vi "SaveConfig.vi"(8 "error in (no error)":errorcluster, 11 "DataLogger in":refnum<class "DataLogger.lvclass">) -> (0 "error out":errorcluster, 3 "DataLogger out":refnum<class "DataLogger.lvclass">)   [LabVIEW 2020, in "DataLogger.lvlib" / "DataLogger.lvclass"]
uses:
  DataLogger.lvclass
  DataLogger.lvclass/DataLogger.ctl
  Hardware Abstraction Layer/Component/GenericActor/GenericActor/GenericActor.lvclass
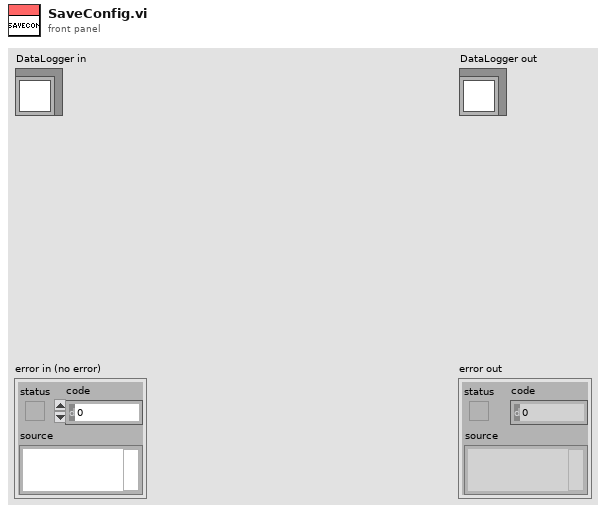
[diagram p1: front panel]
types:
  T1 = typedef "NI_LVConfig.lvlib/Config Data RefNum.ctl" = refnum<k1>
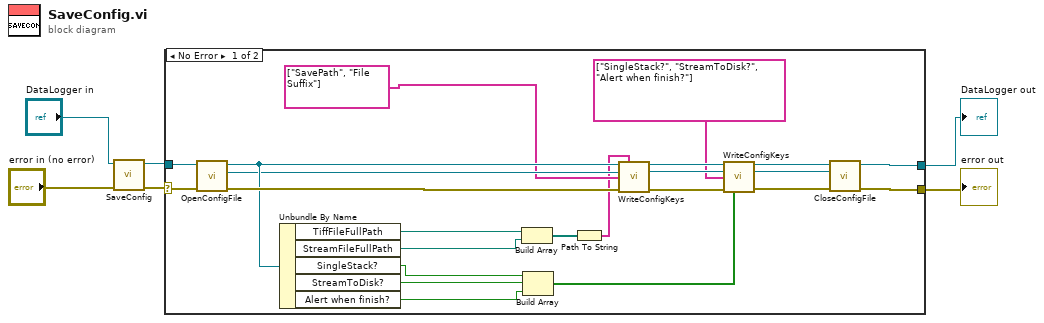
[diagram p0: block diagram]
diagram:
  n1 = call-parent "SaveConfig.vi"("error in (no error)"="error in (no error)", "GRMActor in"="DataLogger in") -> ("error out"=w3:errorcluster, "GRMActor out"=w4:refnum<class "DataLogger.lvclass">)  [unwired: 8 in]
  n2 = case shown="No Error" w3 {
    selector: w3 -> [w29 w30]
    tunnel: [w25 w30] -> w1
    tunnel: [w24 w31] -> w2
    tunnel: w4 -> [w23 w31]
    frame No Error {
      n3 = call-dynamic "OpenConfigFile.vi"("error in (no error)"=w29, "GRMActor in"=w23) -> ("error out"=w26:errorcluster, "refnum"=w21:T1, "GRMActor out"=w22:refnum<class "DataLogger.lvclass">)  [unwired: 7 in]
      n4 = Unbundle By Name(w22) -> ("TiffFileFullPath"=w27:path, "StreamFileFullPath"=w20:path, "SingleStack?"=w19:bool, "StreamToDisk?"=w18:bool, "Alert when finish?"=w17:bool)
      n5 = Build Array(w27, w20) -> (w8:path[])
      n6 = Build Array(w19, w18, w17) -> (w9:bool[])
      n7 = Path To String(path=w8) -> (string=w7:string[])
      n8 = call-dynamic "WriteConfigKeys.vi"("GRMActor in"=w22, "StringValues"=w7, "Config Refnum"=w21, "Keys"=string[] ["SavePath", "File Suffix"] ("Values"), "error in (no error)"=w26) -> ("GRMActor out"=w15:refnum<class "DataLogger.lvclass">, "Config Refnum dup"=w13:T1, "error out"=w28:errorcluster)  [unwired: 8 in]
      n9 = call-dynamic "WriteConfigKeys.vi"("GRMActor in"=w15, "Config Refnum"=w13, "Keys"=string[] ["SingleStack?", "StreamToDisk?", "Alert when finish?"], "error in (no error)"=w28, "BoolValues"=w9) -> ("GRMActor out"=w14:refnum<class "DataLogger.lvclass">, "Config Refnum dup"=w12:T1, "error out"=w16:errorcluster)  [unwired: 8 in]
      n10 = call-dynamic "CloseConfigFile.vi"("error in (no error)"=w16, "refnum"=w12, "GRMActor in"=w14) -> ("error out"=w25:errorcluster, "GRMActor out"=w24:refnum<class "DataLogger.lvclass">)  [unwired: 7 in]
    }
    frame Error {
    }
  }
  "error out" <- w1
  "DataLogger out" <- w2
